vi "Log Data.vi"(8 "error in":errorcluster, 10 "data for logging":T1, 11 "module reference in":T2) -> (0 "error out":errorcluster, 3 "module reference out":T2)   [LabVIEW 2017, in "WinHost.lvlib"]
uses:
  WinHost.lvlib
  Private TypeDefs/Module Reference.ctl
  Global TypeDefs/Registered Modules.ctl
  Private TypeDefs/Module Queues.ctl
  Private TypeDefs/Message Queue Element.ctl
  Public TypeDefs/Messages.ctl
  Private TypeDefs/STM Queue Element.ctl
  Private TypeDefs/Module Notifiers.ctl
  Private TypeDefs/Dummy Notifier.ctl
  mypam/Public TypeDefs/Data for Logging.ctl
  mypam/myPAM.lvlib
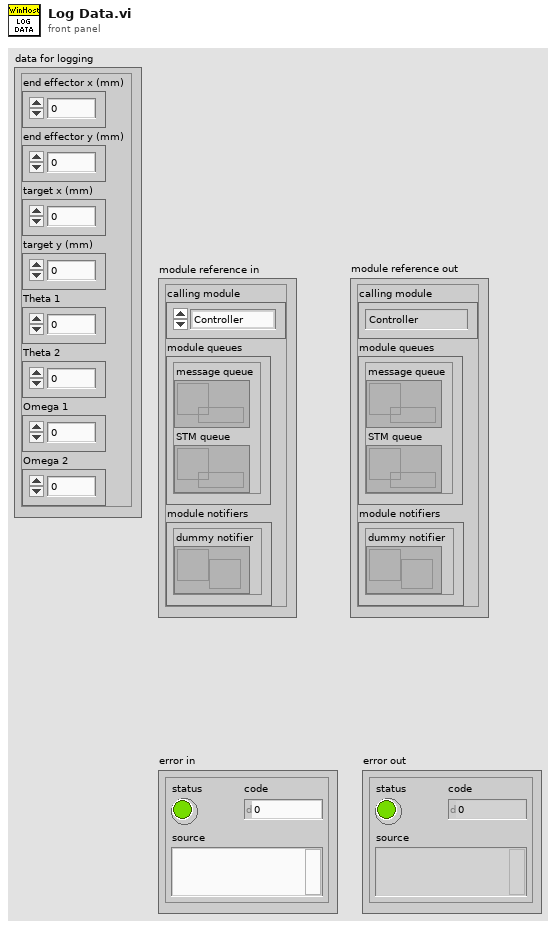
[diagram p1: front panel]
types:
  T1 = typedef "myPAM.lvlib/Data for Logging.ctl" = cluster{"end effector x (mm)":dbl, "end effector y (mm)":dbl, "target x (mm)":dbl, "target y (mm)":dbl, "Theta 1":dbl, "Theta 2":dbl, "Omega 1":dbl, "Omega 2":dbl}
  T2 = typedef "WinHost.lvlib/Module Reference.ctl" = cluster{"calling module":T3, "module queues":T4, "module notifiers":T5}
  T3 = typedef "Registered Modules.ctl" = enum16{"Controller", "DAQ", "Error Handler", "Game", "myPAM", "WinHost", "Logger"}
  T4 = typedef "WinHost.lvlib/Module Queues.ctl" = cluster{"message queue":refnum<queue>, "STM queue":refnum<queue>}
  T5 = typedef "WinHost.lvlib/Module Notifiers.ctl" = cluster{"dummy notifier":refnum<notifier>}
  T6 = typedef "WinHost.lvlib/STM Queue Element.ctl" = cluster{"name":string, "data":string, "stop":bool}
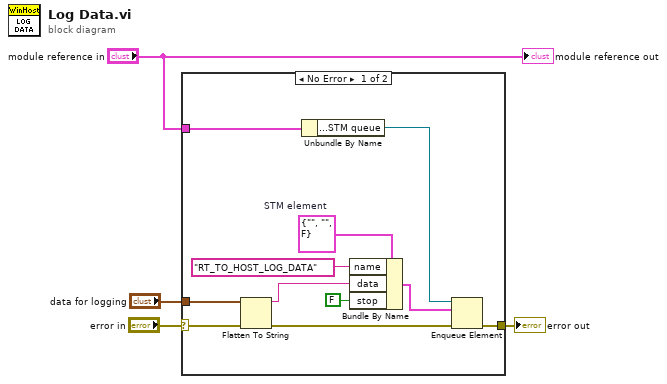
[diagram p0: block diagram]
diagram:
  n1 = case shown="No Error" "error in" {
    selector: "error in" -> [w9 w16]
    tunnel: [w14 w16] -> w4
    tunnel: "module reference in" -> [w15 _]
    tunnel: "data for logging" -> [w5 _]
    frame No Error {
      w12 = T6 {"name"="", "data"="", "stop"=FALSE}  # STM element
      n2 = Flatten To String(anything=w5, error in (no error)=w9) -> (data string=w8:string, error out=w7:errorcluster)  [unwired: 2 in, 1 out]
      n3 = Unbundle By Name(w15) -> ("module queues.STM queue"=w13:refnum<queue>)
      n4 = Bundle By Name(cluster=w12, "name"="RT_TO_HOST_LOG_DATA", "data"=w8, "stop"=FALSE) -> (w11:T6)
      n5 = Enqueue Element(queue=w13, element=w11, error in (no error)=w7) -> (error out=w14:errorcluster)  [unwired: 1 in, 2 out]
    }
    frame Error {
    }
  }
  "error out" <- w4
  "module reference out" <- "module reference in"
